vi "ExposeRegisterStaticReference.vi"(10 "Static refrence ID":string, 11 "Expose Info":T1) -> (3 "Expose Info out":T1)   [LabVIEW 2017]
uses:
  ExposeInfo.ctl
  C:/Code/CMCryoSysCode/Expose/COM/CSCom/CSCom/bin/Release/CSCom.dll
  COM/CSCom/CSCom/bin/Release/CSCom.dll
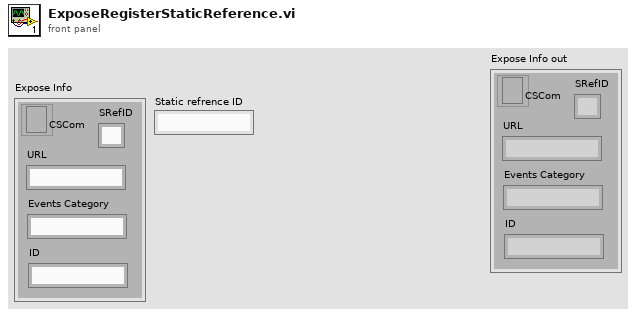
[diagram p1: front panel]
types:
  T1 = typedef "ExposeInfo.ctl" = cluster{"CSCom":refnum<k24>, "URL":string, "Events Category":string, "ID":string, "SRefID":string}
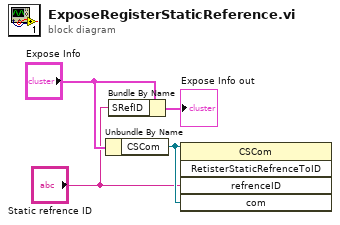
[diagram p0: block diagram]
diagram:
  n1 = Unbundle By Name("Expose Info") -> ("CSCom"=w4:refnum<k24>)
  n2 = Bundle By Name(cluster="Expose Info", "SRefID"="Static refrence ID") -> (→"Expose Info out":T1)
  n3 = invoke class="CSCom" method="RetisterStaticRefrenceToID"(reference=w4, "refrenceID"="Static refrence ID", "com"=w4) -> ()  [unwired: 2 in, 5 out]
